vi "FourFlippingCoins.vi"() -> ()   [LabVIEW 2014]
panel:
  out "Histogram":dynamicdata(graph)
  in  "Number of Trials":dbl
  out "Number of Heads":dbl
  out "Coin 4":bool
  out "Coin 3":bool
  out "Coin 2":bool
  out "Coin 1":bool
  # "Description of Block Diagram Components:\n\n-Number of Trials: The  \"number of trials\" input on the front panel is \n                                   fed into the for loop counter, so that the for loop\n                                   runs that amount of times to generate that amount\n                                   of flip simulations.\n\n-Decision Constant: After the random number generators generate a zero \n                                     or a one, they are fed into a greater or equal then \n                                     comparator. The Decision Constant is the number that\n                                     is compared with the randomly generated number to \n                                     decide whether the simulation outputted a head or tail.\n\n-Heads or Tails Indication: The comparators output a true or false boolean\n                                                result. The heads or tails indications use these\n                                                boolean results to facilitate the coin lights on \n                                                the front panel. If the boolean result is true, the\n                                                indicator triggers the light for that respective coin\n                                                on the front panel, indicating a heads condition. \n\nBoolean to Integer: These four devices, one for each coin result, convert the\n                                   boolean true or false value to a numerical one or zero. \n\nTrial Head Counter: Now that the coin flip results are in numerical form,  they\n                                    can be analyzed as a set of data. The Trial Head Counter\n                                    adds up the results of the boolean to numerical conversions,\n                                    and the  sum of this number is the number of heads. This \n                                    value is exported to a visual counter on the front panel, as\n                                    well as going out of the for loop to build an array. This\n                                    creates a 1D array, the length of which is decided by the\n                                    number of trials, which is outputted to the histogram for\n                                    data analysis."
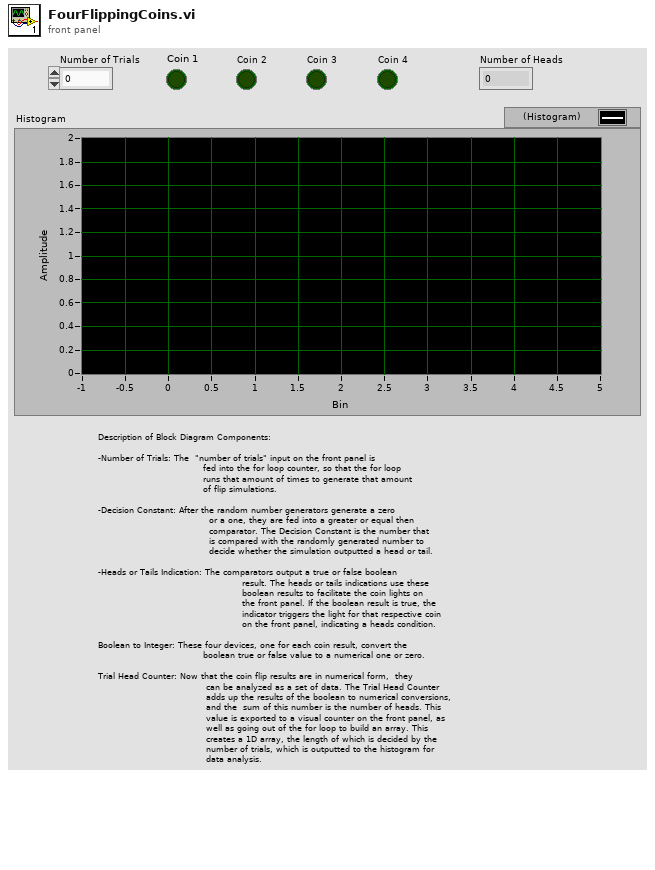
[diagram p1: front panel]
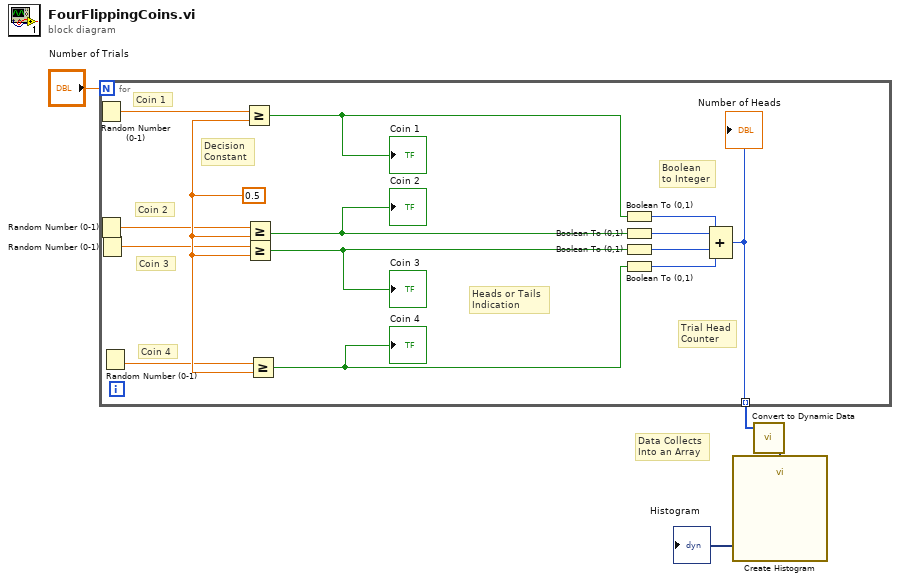
[diagram p0: block diagram]
diagram:
  # "Data Collects\nInto an Array"
  n1 = for {
    N: "Number of Trials" -> [_]
    tunnel: [w5] -> w1 mode=indexing
    w9 = 0.5
    # "Coin 4"
    # "Coin 3"
    # "Coin 2"
    # "Coin 1"
    # "Trial Head\nCounter"
    # "Heads or Tails\nIndication"
    # "Boolean\nto Integer"
    # "Decision \nConstant"
    n2 = Random Number (0-1)() -> (number: 0 to 1=w10:dbl)
    n3 = Random Number (0-1)() -> (number: 0 to 1=w6:dbl)
    n4 = Random Number (0-1)() -> (number: 0 to 1=w7:dbl)
    n5 = Random Number (0-1)() -> (number: 0 to 1=w8:dbl)
    n6 = Greater Or Equal?(x=w10, y=w9) -> (x >= y?=w15:bool)
    "Coin 1" <- w15
    n7 = Greater Or Equal?(x=w6, y=w9) -> (x >= y?=w16:bool)
    "Coin 2" <- w16
    n8 = Greater Or Equal?(x=w7, y=w9) -> (x >= y?=w17:bool)
    "Coin 3" <- w17
    n9 = Greater Or Equal?(x=w8, y=w9) -> (x >= y?=w18:bool)
    "Coin 4" <- w18
    n10 = Boolean To (0,1)(Boolean=w15) -> (0, 1=w11:i16)
    n11 = Boolean To (0,1)(Boolean=w16) -> (0, 1=w12:i16)
    n12 = Boolean To (0,1)(Boolean=w17) -> (0, 1=w13:i16)
    n13 = Boolean To (0,1)(Boolean=w18) -> (0, 1=w14:i16)
    n14 = Compound Arithmetic op=ADD(w11, w12, w13, w14) -> (w5:i16)
    "Number of Heads" <- w5
  }
  n15 = call "Convert to Dynamic Data"("Array"=w1) -> ("Dynamic Data Type"=w3:dynamicdata)  [unwired: 3 in]
  n16 = call "Create Histogram"("Signal"=w3) -> ("Histogram"=→"Histogram":dynamicdata)  [unwired: 9 in, 1 out]
